vi "MGCC_MdlMgmt_Data-read-from-txt.vi"(10 "file path (use dialog)":path) -> (2 "text":string)   [LabVIEW 2016]
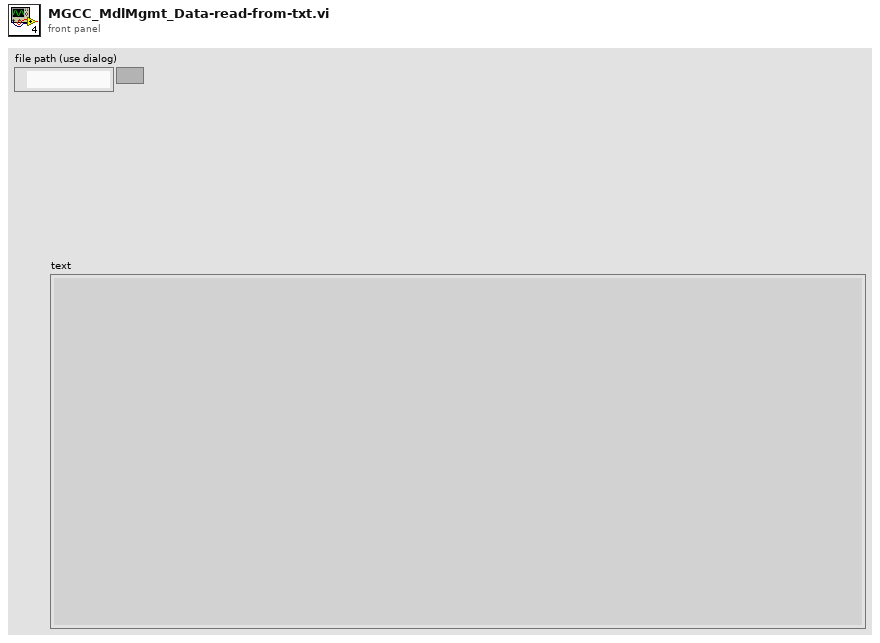
[diagram p1: front panel]
types:
  T1 = enum16{"open", "replace", "create", "open or create", "replace or create", "replace or create with confirmation"}
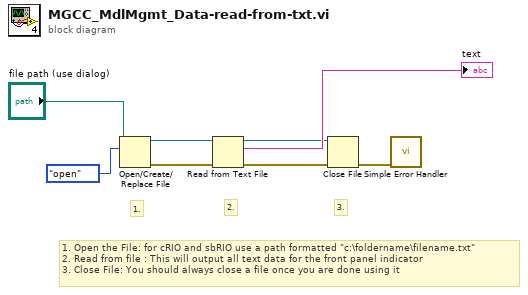
[diagram p0: block diagram]
diagram:
  # "1. Open the File: for cRIO and sbRIO use a path formatted \"c:\\foldername\\filename.txt\"\n2. Read from file : This will output all text data for the front panel indicator\n3. Close File: You should always close a file once you are done using it"
  # "3."
  # "2."
  # "1."
  n1 = Open/Create/Replace File(file path (use dialog)="file path (use dialog)", operation (0:open)=T1."open") -> (refnum out=w3:refnum<file>, error out=w2:errorcluster)  [unwired: 4 in, 1 out]
  n2 = Read from Text File(file (use dialog)=w3, error in=w2) -> (refnum out=w6:refnum<file>, text=→"text":string, error out=w7:errorcluster)  [unwired: 2 in, 1 out]
  n3 = Close File(refnum=w6, error in=w7) -> (error out=w5:errorcluster)  [unwired: 1 out]
  n4 = call <vilib>:"Simple Error Handler.vi"("error in (no error)"=w5) -> ()  [unwired: 4 in, 5 out]
